vi "Initialize Inline Buffer.vi"(8 "error in (no error)":errorcluster, 9 "channel count":u64, 10 "first channel offset":u64, 11 "Framework in":refnum<class "VeriStand DSF.Framework.lvclass">) -> (0 "error out":errorcluster, 2 "Buffer":refnum<class "Double Pointer.lvclass">, 3 "Framework out":refnum<class "VeriStand DSF.Framework.lvclass">)   [LabVIEW 2017, in "Data Sharing Framework Engine.lvlib" / "VeriStand DSF.Framework.lvclass"]
uses:
  VeriStand DSF.Framework.lvclass
  Builds/Current/Data Sharing Framework Core/Data Sharing Framework Core.lvlibp/Engine/Internal/Memory/Double Pointer/Double Pointer.lvclass
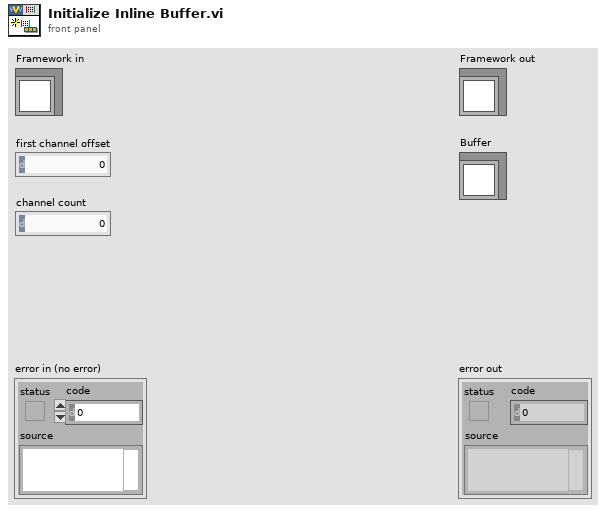
[diagram p1: front panel]
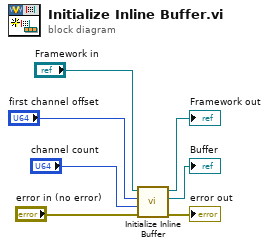
[diagram p0: block diagram]
diagram:
  n1 = call-dynamic "Initialize Inline Buffer.vi"("error in (no error)"="error in (no error)", "channel count"="channel count", "first channel offset"="first channel offset", "Framework in"="Framework in") -> ("error out"=→"error out":errorcluster, "Buffer"=→"Buffer":refnum<class "Double Pointer.lvclass">, "Framework out"=→"Framework out":refnum<class "VeriStand DSF.Framework.lvclass">)  [unwired: 5 in]
